vi "Command Information.vi"() -> (0 "Variant":variant)   [LabVIEW 2018]
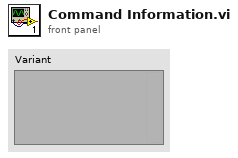
[diagram p1: front panel]
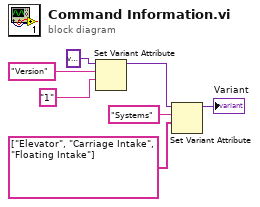
[diagram p0: block diagram]
diagram:
  n1 = Set Variant Attribute(Variant=variant, name="Version", value="1" ("name")) -> (Variant out=w5:variant)  [unwired: 1 in, 2 out]
  n2 = Set Variant Attribute(Variant=w5, name="Systems", value=string[] ["Elevator", "Carriage Intake", "Floating Intake"]) -> (Variant out=→"Variant":variant)  [unwired: 1 in, 2 out]
